vi "Format Num Array Cmd.vi"(4 "Command":T1[](array[typedef])) -> (7 "String":string)   [LabVIEW 2020, in "Volatus.lvlib" / "Module.lvclass"]
uses:
  Module.lvclass
  Module.lvclass/Module.ctl
  messages/CmdAnalog/Data.ctl
  messages/CmdAnalog/CmdAnalog.lvlib
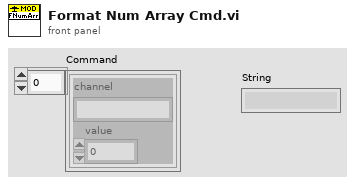
[diagram p1: front panel]
types:
  T1 = typedef "CmdAnalog.lvlib/Data.ctl" = cluster{"channel":string, "value":dbl}
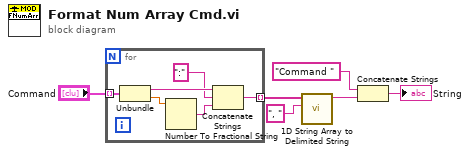
[diagram p0: block diagram]
diagram:
  n1 = for {
    tunnel: "Command" -> [w12] mode=indexing
    tunnel: [w9] -> w5 mode=indexing
    n2 = Unbundle(w12) -> ("channel"=w11:string, "value"=w8:dbl)
    n3 = Number To Fractional String(number=w8) -> (F-format string=w7:string)  [unwired: 3 in]
    n4 = Concatenate Strings(w11, ":" ("string"), w7) -> (w9:string)
  }
  n5 = call <vilib>:"1D String Array to Delimited String.vi"("delimiter"=", ", "string array"=w5) -> ("delimited string"=w3:string)  [unwired: 9 in]
  n6 = Concatenate Strings("Command " ("string"), w3) -> (→"String":string)
